vi "Fusion Multicast Receiver-Sender.vi"() -> ()   [LabVIEW 2015]
doc: "Creates a read-only UDP multicast session and receives data on the specified port."
uses:
  <vilib>/Utility/tcp.llb/UDP Multicast Read-Only Open.vi
panel:
  in  "Stop 2":bool
  out "Current Data Value":dbl
  out "Sensor Fusion Data":dbl(graph)
  in  "Stop":bool
  # "Overview: Demonstrates the use of the UDP functions to connect to a UDP multicast session and receive data.\nInstructions:\n1. Ensure UDP Multicast - xbox_listener.cpp is already running.\n2. Run the VI.\n3. Click Stop to stop the VI."
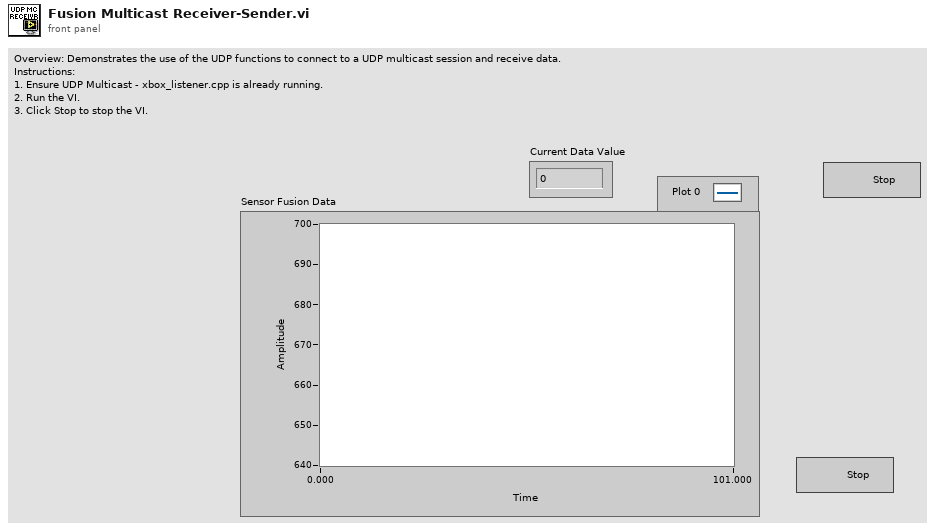
[diagram p1: front panel]
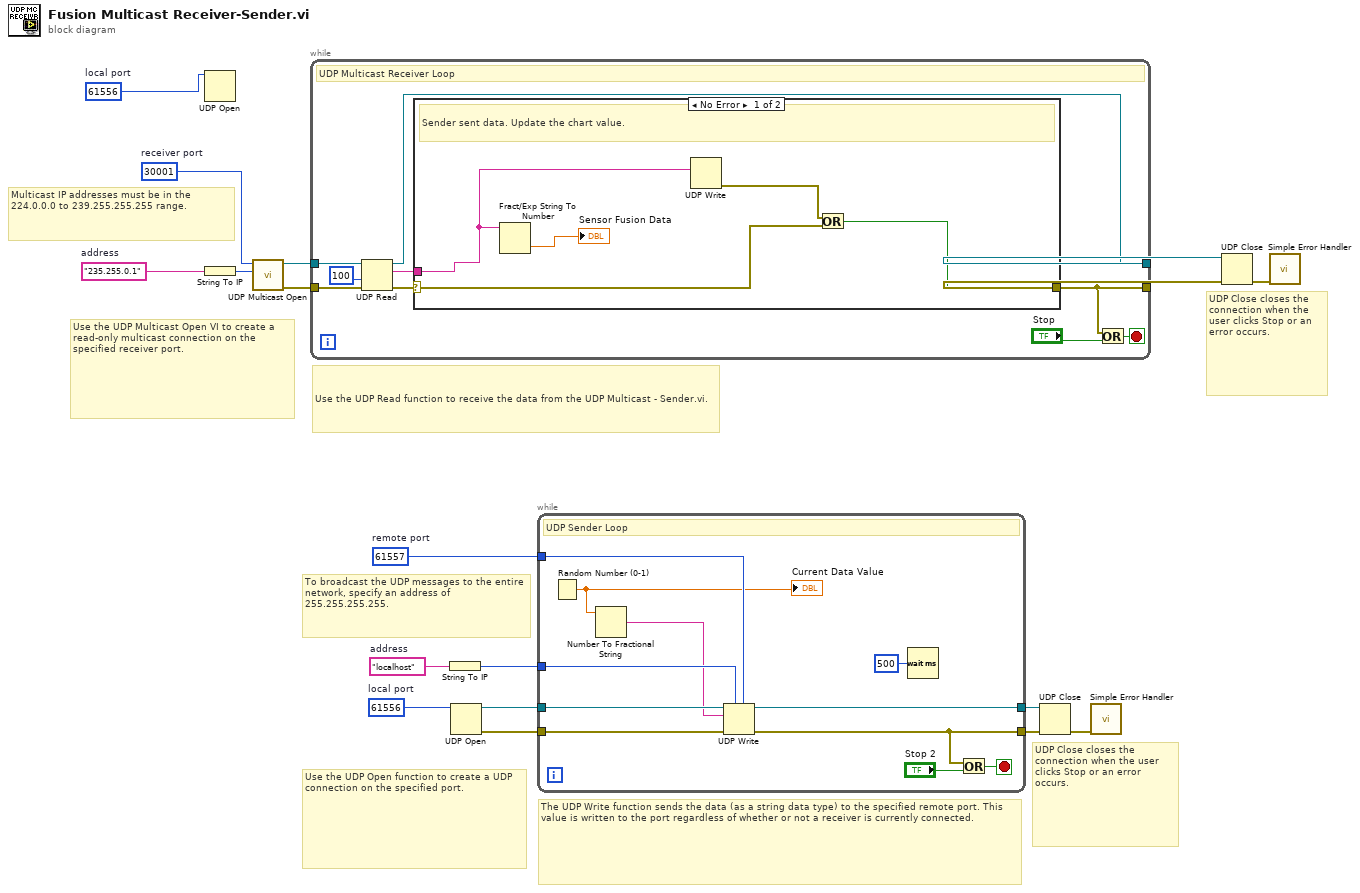
[diagram p0: block diagram]
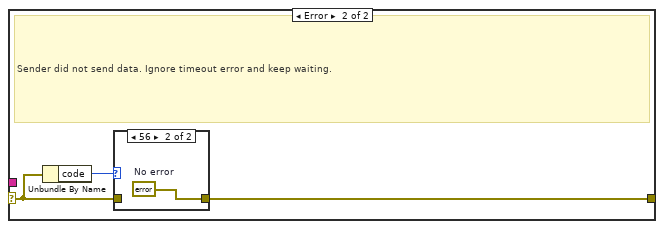
[diagram p2: hidden frame]
diagram:
  w1 = u16 61556  # local port
  w2 = u16 61557  # remote port
  w3 = u16 61556  # local port
  w8 = "localhost"  # address
  w12 = u16 30001  # receiver port
  w17 = "235.255.0.1"  # address
  # "To broadcast the UDP messages to the entire network, specify an address of 255.255.255.255."
  # "UDP Close closes the connection when the user clicks Stop or an error occurs."
  # "The UDP Write function sends the data (as a string data type) to the specified remote port. This value is written to the port regardless of whether or not a receiver is currently connected."
  # "Use the UDP Open function to create a UDP connection on the specified port."
  # "UDP Close closes the connection when the user clicks Stop or an error occurs."
  # "Use the UDP Multicast Open VI to create a read-only multicast connection on the specified receiver port."
  # "Multicast IP addresses must be in the 224.0.0.0 to 239.255.255.255 range."
  # "Use the UDP Read function to receive the data from the UDP Multicast - Sender.vi."
  n1 = UDP Open(11:w1) -> ()  [unwired: 4 in, 3 out]
  n2 = String To IP(1:w17) -> (0:w11:u32)
  n3 = call-poly <vilib>:"UDP Multicast Open.vi"("multicast addr"=w11, "port"=w12) -> ("error out"=w14:errorcluster, "connection ID"=w13:refnum<k16>)  [unwired: 7 in, 1 out]
  n4 = while {
    tunnel: w13 -> [w27]
    tunnel: [w19] -> w18
    tunnel: w14 -> [w24]
    tunnel: [w20] -> w15
    stop <- w25 stop-if-true
    # "UDP Multicast Receiver Loop"
    n5 = UDP Read(connection ID=w27, timeout ms (25000)=100, 8:w24) -> (data out=w22:string, error out=w21:errorcluster, 3:w19:refnum<k16>)  [unwired: 3 out]
    n6 = case shown="No Error" w21 {
      selector: w21 -> [w29 w34]
      tunnel: w22 -> [w31 _]
      tunnel: [w28 w33] -> w20
      frame No Error {
        # "Sender sent data. Update the chart value."
        n7 = Fract/Exp String To Number(string=w31) -> (number=→"Sensor Fusion Data":dbl)  [unwired: 3 in, 1 out]
        n8 = UDP Write(data in=w31) -> (error out=w30:errorcluster)  [unwired: 5 in, 1 out]
        n9 = Or(x=w30, y=w29) -> (x .or. y?=w28:bool)
      }
      frame Error {
        # "Sender did not send data. Ignore timeout error and keep waiting."
        n10 = Unbundle By Name(w34) -> ("code"=w35:i32)
        n11 = case shown="56" w35 {
          tunnel: w34 -> [w36 _]
          tunnel: [w36 w37] -> w33
          frame Default {
          }
          frame 56 {
            w37 = errorcluster {"status"=FALSE, "code"=0, "source"=""}  # No error
          }
        }
      }
    }
    n12 = Or(x=w20, y="Stop") -> (x .or. y?=w25:bool)
  }
  n13 = String To IP(1:w8) -> (0:w6:u32)
  n14 = UDP Open(11:w3) -> (port=w5:refnum<k16>, 0:w4:errorcluster)  [unwired: 4 in, 1 out]
  n15 = while {
    tunnel: [w43] -> w9
    tunnel: w5 -> [w48]
    tunnel: w4 -> [w47]
    tunnel: [w44] -> w10
    tunnel: w6 -> [w42]
    tunnel: w2 -> [w39]
    stop <- w46 stop-if-true
    # "UDP Sender Loop"
    n16 = Random Number (0-1)() -> (number: 0 to 1=w38:dbl)
    "Current Data Value" <- w38
    n17 = Number To Fractional String(number=w38) -> (F-format string=w40:string)  [unwired: 3 in]
    n18 = UDP Write(address=w42, port or service name=w39, connection ID=w48, data in=w40, 8:w47) -> (error out=w43:errorcluster, 3:w44:refnum<k16>)  [unwired: 1 in]
    n19 = Wait (ms)(milliseconds to wait=u32 500) -> ()  [unwired: 1 out]
    n20 = Or(x=w43, y="Stop 2") -> (x .or. y?=w46:bool)
  }
  n21 = UDP Close(connection ID=w10, 8:w9) -> (error out=w7:errorcluster)  [unwired: 1 out]
  n22 = call <vilib>:"Simple Error Handler.vi"("error in (no error)"=w7) -> ()  [unwired: 4 in, 5 out]
  n23 = UDP Close(connection ID=w18, 8:w15) -> (error out=w16:errorcluster)  [unwired: 1 out]
  n24 = call <vilib>:"Simple Error Handler.vi"("error in (no error)"=w16) -> ()  [unwired: 1 in, 8 out]
